vi "Perform Action.vi"(8 "error in":errorcluster, 10 "Input":variant, 11 "DO DAQmx PWM Fixed Freq in":refnum<class "DO DAQmx Fixed Freq PWM CFG Simulated.lvclass">) -> (0 "error out":errorcluster, 2 "Output":variant, 3 "DO DAQmx PWM Fixed Freq out":refnum<class "DO DAQmx Fixed Freq PWM CFG Simulated.lvclass">)   [LabVIEW 2024, in "DAQmx Simulated CFGs.lvlib" / "DO DAQmx Fixed Freq PWM CFG Simulated.lvclass"]
uses:
  DO DAQmx Fixed Freq PWM CFG Simulated.lvclass
  DO DAQmx Fixed Freq PWM CFG/DO DAQmx Fixed Freq PWM CFG.lvclass
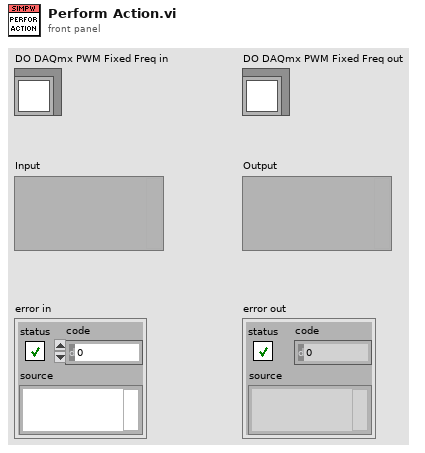
[diagram p1: front panel]
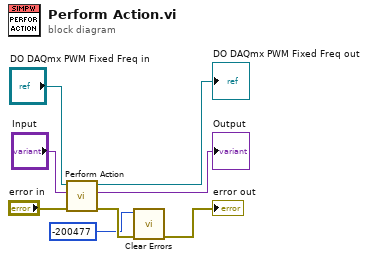
[diagram p0: block diagram]
diagram:
  n1 = call-parent "Perform Action.vi"("error in"="error in", "Input"="Input", "DO DAQmx Fixed Freq PWM CFG in"="DO DAQmx PWM Fixed Freq in") -> ("error out"=w8:errorcluster, "Output"=→"Output":variant, "DO DAQmx Fixed Freq PWM CFG out"=→"DO DAQmx PWM Fixed Freq out":refnum<class "DO DAQmx Fixed Freq PWM CFG Simulated.lvclass">)  [unwired: 6 in]
  n2 = call <vilib>:"Clear Errors.vi"("error in (no error)"=w8, "specific error code to clear (0: all)"=-200477) -> ("error out"=→"error out":errorcluster)  [unwired: 4 in, 1 out]
